vi "Get Start of Whitespace Pixel Number.vi"(11 "Positive Transitions":bool[](array[boolean])) -> (3 "Row/Col where whitespace starts":i32[](array[numeric]))   [LabVIEW 2018, in "Image Management.lvlib"]
uses:
  Image Management.lvlib
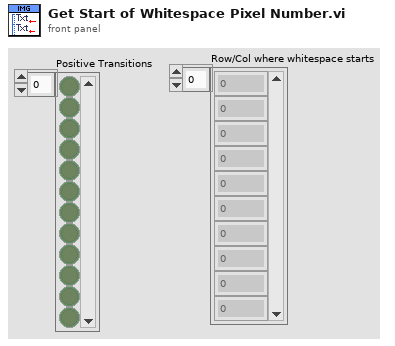
[diagram p1: front panel]
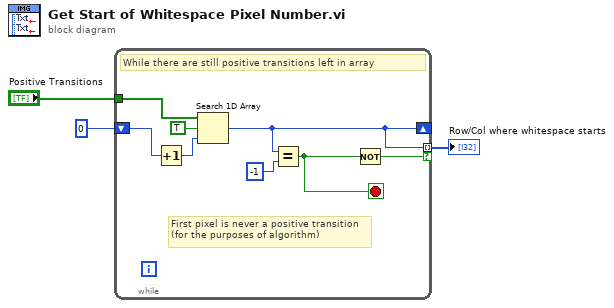
[diagram p0: block diagram]
diagram:
  n1 = while {
    tunnel: "Positive Transitions" -> [w11]
    shift-right: [w7] -> _
    shift-left: 0 ("index of element") -> [w9]
    tunnel: [w7] -> w3 mode=indexing if=w5
    stop <- w4 stop-if-true
    # "First pixel is never a positive transition\n(for the purposes of algorithm)"
    # "While there are still positive transitions left in array"
    n2 = Increment(x=w9) -> (x+1=w8:i32)
    n3 = Search 1D Array(1D array=w11, element=TRUE, start index (0)=w8) -> (index of element=w7:i32)
    n4 = Equal?(x=w7, y=-1) -> (x = y?=w4:bool)
    n5 = Not(x=w4) -> (.not. x?=w5:bool)
  }
  "Row/Col where whitespace starts" <- w3
